vi "ParseEventJson.vi"(8 "Error In":errorcluster, 11 "EventJson":string) -> (0 "Error Out":errorcluster, 2 "Type":string, 3 "JSON Tree Out":variant)   [LabVIEW 2017, in "LiteAgentSDK.lvlib"]
uses:
  LiteAgentSDK.lvlib
  <vilib>/LVH/i3 JSON/JSON Parsing/Get Object Parameter Files/Get Object Parameter - String.vi
  <vilib>/LVH/i3 JSON/i3-json.lvlib
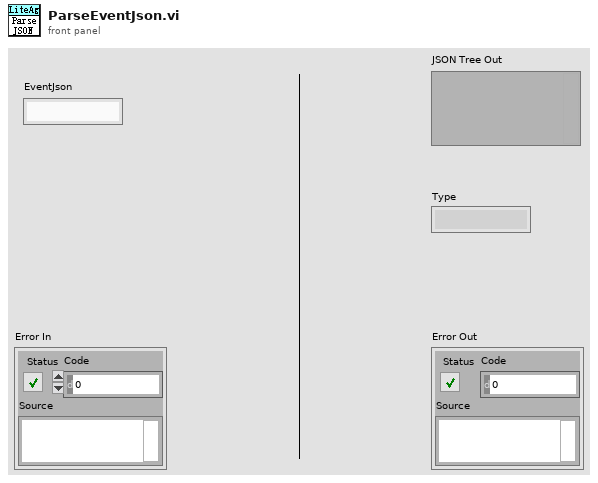
[diagram p1: front panel]
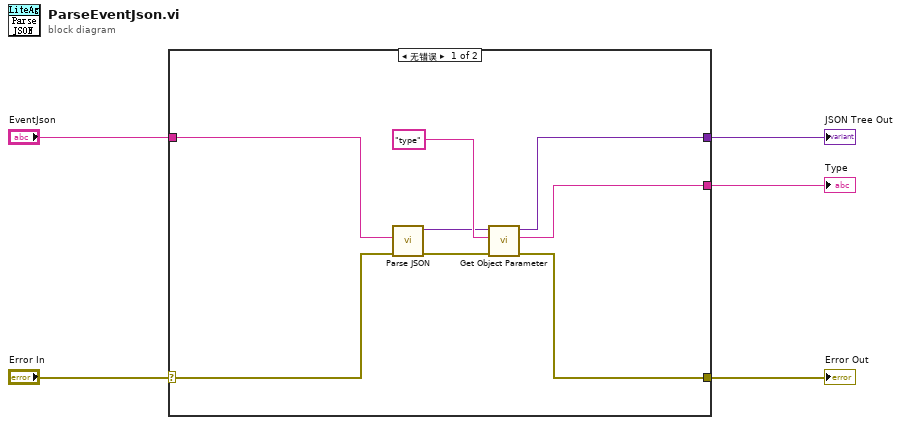
[diagram p0: block diagram]
diagram:
  n1 = case shown="无错误" "Error In" {
    selector: "Error In" -> [w13 w14]
    tunnel: [w8 w14] -> w4
    tunnel: "EventJson" -> [w12 _]
    tunnel: [w7 _] -> w2
    tunnel: [w6 _] -> w1
    frame No Error {
      n2 = call <vilib>:"Parse JSON.vi"("error in (no error)"=w13, "JSON String"=w12) -> ("error out"=w9:errorcluster, "JSON Tree"=w10:variant)  [unwired: 6 in, 2 out]
      n3 = call-poly <vilib>:"Get Object Parameter.vi"("error in (no error)"=w9, "Parameter Name"="type", "JSON Tree In (JSON Object)"=w10) -> ("error out"=w8:errorcluster, "String Value"=w7:string, "JSON Tree Out Passthrough"=w6:variant)  [unwired: 5 in, 1 out]
    }
    frame Error {
    }
  }
  "Error Out" <- w4
  "Type" <- w2
  "JSON Tree Out" <- w1
